vi "Write Report.vi"(8 "error in (no error)":errorcluster, 10 "Resource In":variant, 11 "Analyze Results q-Factor in":refnum<class "Analyze Results q-Factor.lvclass">) -> (0 "error out":errorcluster, 2 "Resource Out":variant, 3 "Analyze Results q-Factor out":refnum<class "Analyze Results q-Factor.lvclass">)   [LabVIEW 2014, in "Analyze Results q-Factor.lvclass"]
uses:
  Analyze Results q-Factor.lvclass
  <vilib>/Utility/config.llb/Config Data RefNum.ctl
  Results Base/Analyze Results Base.lvclass/Analyze Results Base.ctl
  Analyze Results q-Factor.lvclass/Analyze Results q-Factor.ctl
  Results Base/Read Section.vi
  <vilib>/Utility/config.llb/Write Key (Double).vi
  <vilib>/Utility/config.llb/NI_LVConfig.lvlib
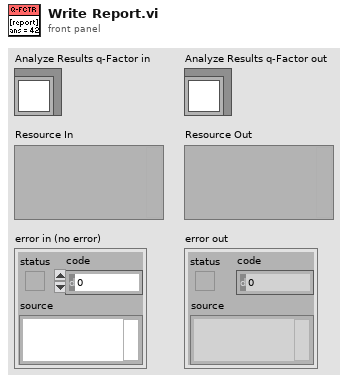
[diagram p1: front panel]
types:
  T1 = typedef "NI_LVConfig.lvlib/Config Data RefNum.ctl" = refnum<k1>
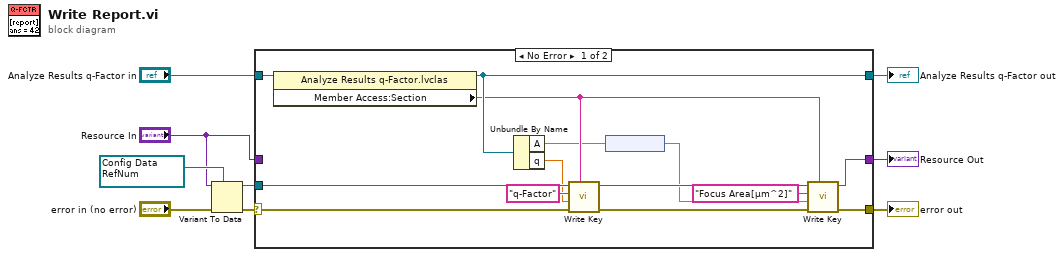
[diagram p0: block diagram]
diagram:
  w7 = T1 refnum items=["config data"] ("refnum")
  n1 = Variant To Data(error in="error in (no error)", type=w7, Variant="Resource In") -> (data=w8:T1, error out=w9:errorcluster)
  n2 = case shown="No Error" w9 {
    selector: w9 -> [w19 w25]
    tunnel: w8 -> [w20 _]
    tunnel: "Analyze Results q-Factor in" -> [w23 w24]
    tunnel: [w22 w24] -> w1
    tunnel: [w17 w26] -> w3
    tunnel: [w16 w25] -> w2
    tunnel: "Resource In" -> [_ w26]
    frame No Error {
      n3 = property class="Analyze Results q-Factor.lvclas"(reference=w23) -> (reference out=w22:refnum<class "Analyze Results q-Factor.lvclass">, "Member Access:Section"=w18:string)  [unwired: 1 in, 1 out]
      n4 = Unbundle By Name(w22) -> ("A"=w12:dbl[unit], "q"=w13:dbl)
      n5 = call-poly <vilib>:"Write Key.vi"("section"=w18, "error in (no error)"=w19, "value"=w13, "key"="q-Factor", "refnum"=w20) -> ("error out"=w15:errorcluster, "refnum out"=w21:T1)  [unwired: 4 in, 1 out]
      n6 = node(w12) -> (w11:dbl)
      n7 = call-poly <vilib>:"Write Key.vi"("section"=w18, "error in (no error)"=w15, "value"=w11, "key"="Focus Area[µm^2]", "refnum"=w21) -> ("error out"=w16:errorcluster, "refnum out"=w17:T1)  [unwired: 4 in, 1 out]
    }
    frame Error {
    }
  }
  "error out" <- w2
  "Analyze Results q-Factor out" <- w1
  "Resource Out" <- w3
